vi "createLabelsFromSelection.vi"(1 "log_from":string, 2 "Controls[]":refnum<vi>[](array[refnum])) -> (0 "labels_to_log":string[](array[string]))   [LabVIEW 2017]
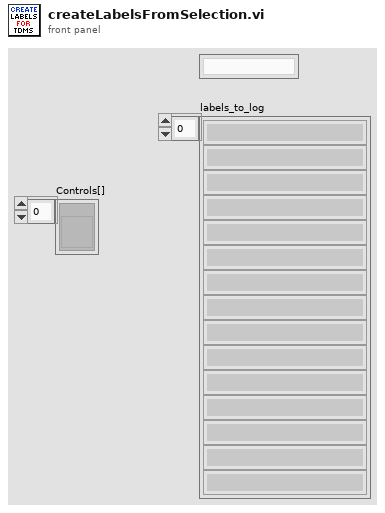
[diagram p1: front panel]
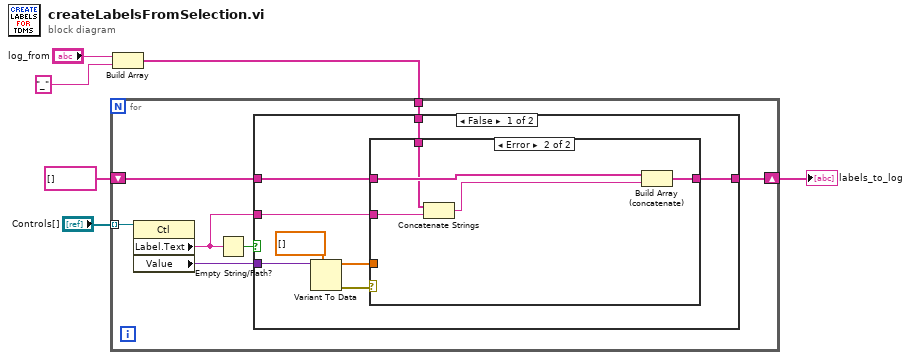
[diagram p0: block diagram]
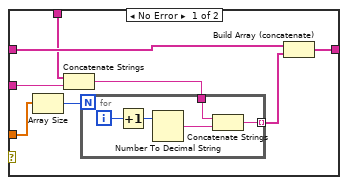
[diagram p2: hidden frame]
diagram:
  n1 = Build Array("log_from", "_") -> (w1:string[])
  n2 = for {
    tunnel: "Controls[]" -> [w10] mode=indexing
    shift-right: [w13] -> w5
    shift-left: string[] [] -> [w12]
    tunnel: w1 -> [w11]
    n3 = property class="Ctl"(reference=w10) -> ("Label.Text"=w8:string, "Value"=w9:variant)  [unwired: 1 in, 2 out]
    n4 = Empty String/Path?(string/path=w8) -> (empty?=w7:bool)
    n5 = case shown="False" w7 {
      tunnel: w9 -> [w19 _]
      tunnel: [w18 w40] -> w13
      tunnel: w12 -> [w16 w40]
      tunnel: w11 -> [w15 _]
      tunnel: w8 -> [w14 _]
      frame False {
        n6 = Variant To Data(type=dbl[] [], Variant=w19) -> (data=w17:dbl[], error out=w20:errorcluster)  [unwired: 1 in]
        n7 = case shown="Error" w20 {
          tunnel: [w29 w38] -> w18
          tunnel: w17 -> [w28 _]
          tunnel: w16 -> [w26 w39]
          tunnel: w14 -> [w23 w37]
          tunnel: w15 -> [w24 w35]
          frame No Error {
            n8 = Array Size(array=w28) -> (size(s)=w27:i32)
            n9 = Concatenate Strings(w24, w23) -> (w22:string)
            n10 = for {
              N: w27 -> [_]
              tunnel: [w34] -> w25 mode=indexing
              tunnel: w22 -> [w30]
              i -> [w33]
              n11 = Increment(x=w33) -> (x+1=w32:i32)
              n12 = Number To Decimal String(number=w32) -> (decimal integer string=w31:string)  [unwired: 1 in]
              n13 = Concatenate Strings(w30, w31) -> (w34:string)
            }
            n14 = Build Array (concatenate)(w26, w25) -> (w29:string[])
          }
          frame Error {
            n15 = Concatenate Strings(w35, w37) -> (w36:string)
            n16 = Build Array (concatenate)(w39, w36) -> (w38:string[])
          }
        }
      }
      frame True {
      }
    }
  }
  "labels_to_log" <- w5
